vi "Protocol Read.vi"(8 "error in (no error)":errorcluster, 9 "timeout":i32=10000, 10 "bytes to read":i32, 11 "protocol layer in":refnum<class "Serial Slave.lvclass">) -> (0 "error out":errorcluster, 1 "timed out?":bool, 2 "data":u8[](array[numeric]), 3 "protocol layer out":refnum<class "Serial Slave.lvclass">)   [LabVIEW 2017, in "SubVIs.lvlib" / "Serial Slave.lvclass"]
doc: "This provides an interface for reading from a network bus."
uses:
  <vilib>/Modbus/subvis/Protocol/Serial/Serial Slave/Serial Slave.lvclass
  <vilib>/Modbus/subvis/Protocol/Serial/Serial Slave/Serial Slave.lvclass/Serial Slave.ctl
  <vilib>/Modbus/subvis/Protocol/Serial/Serial Shared Components/Serial Shared Components.lvlib
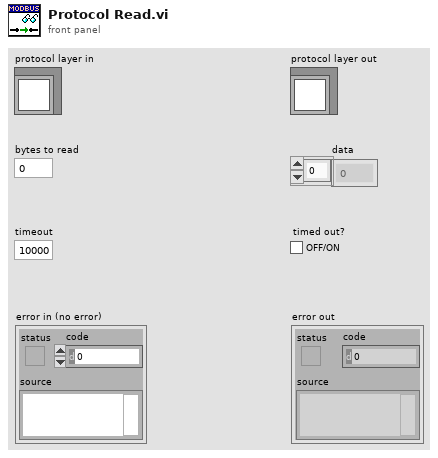
[diagram p1: front panel]
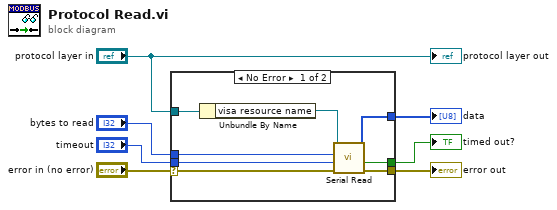
[diagram p0: block diagram]
diagram:
  n1 = case shown="No Error" "error in (no error)" {
    selector: "error in (no error)" -> [w8 w16]
    tunnel: [w15 w16] -> w7
    tunnel: [w14 _] -> w6
    tunnel: "timeout" -> [w13 _]
    tunnel: "bytes to read" -> [w12 _]
    tunnel: "protocol layer in" -> [w11 _]
    tunnel: [w10 _] -> w2
    frame No Error {
      n2 = Unbundle By Name(w11) -> ("visa resource name"=w9:refnum<visa-resource-name>)
      n3 = call <vilib>:"Serial Read.vi"("error in (no error)"=w8, "timeout (ms)"=w13, "bytes to read"=w12, "VISA resource"=w9) -> ("error out"=w15:errorcluster, "timed out?"=w14:bool, "data"=w10:u8[])  [unwired: 5 in]
    }
    frame Error {
    }
  }
  "error out" <- w7
  "data" <- w2
  "timed out?" <- w6
  "protocol layer out" <- "protocol layer in"
